vi "Renishaw-XL80_GetMatTemp.vi"(8 "error in (no error)":errorcluster, 11 "Renishaw-XL80_EMU in":refnum<class "Renishaw-XL80_EMU.lvclass">) -> (0 "error out":errorcluster, 1 "pStatus Array":i32[](array[ring]) items=["SENSOR_OK"=0, "SENSOR_BAD_READING"=1, "SENSOR_FAILED"=2, "SENSOR_NOT_CONNECTED"=4], 2 "Temperature Array":dbl[](array[numeric]), 3 "Renishaw-XL80_EMU out":refnum<class "Renishaw-XL80_EMU.lvclass">)   [LabVIEW 2024, in "Renishaw-XL80_EMU.lvclass"]
doc: "This method disconnects a client from a DX10.\n\nDefinition\nHRESULTGetMatTemp( [in] short nIndex, [out] SENSOR_STATUS_CODES *pStatus, [out, retval] double *pVal);\nParameters\nnIndex\nIdentifies the sensor to be read from. Its value should be in [1..3].\n\npStatus\nA variable that will be set to one of the SENSOR_STATUS_CODES.\n\npVal\nA variable that will be set to the material temperature reading from the specified sensor (in oC).\n\nComments\nThis method will return with an HRESULT of E_INVALIDARG if nIndex is not in [1..3].\n\nIf the client has not connected to the DX10 then the default value (20oC) will be returned and the status will be set to SENSOR_NOT_CONNECTED.\n\nIf the client connected to a DX10 and it subsequently stopped responding, or the EC10 stopped responding then the last values obtained from the EC10 will be returned i.e. the status will not be modified. It is important therefore to monitor both the DX10Status and EC10Status. This is easily done using the _RenishawDX10Events interface.\n\n\nIf the sensor status is SENSOR_NOT_CONNECTED or SENSOR_BAD_READING, then pVal will be set to the last known valid reading.\n\nThe property will normally return an HRESULT of S_OK. However, it will return E_POINTER if the client supplies a null pointer for either pVal or pStatus."
uses:
  Renishaw-XL80_EMU.lvclass
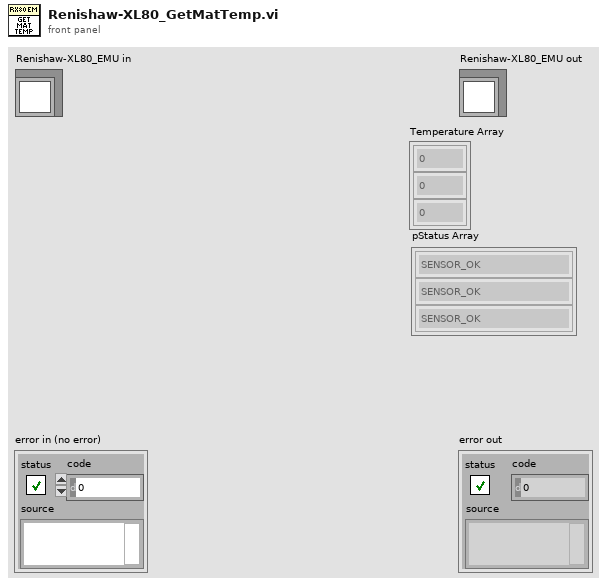
[diagram p1: front panel]
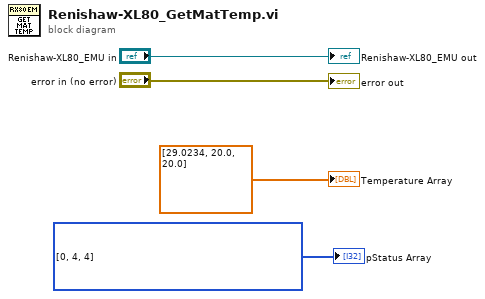
[diagram p0: block diagram]
diagram:
  w1 = i32[] [0, 4, 4] items=["SENSOR_OK"=0, "SENSOR_BAD_READING"=1, "SENSOR_FAILED"=2, "SENSOR_NOT_CONNECTED"=4] ("pStatus Array")
  "error out" <- "error in (no error)"
  "Renishaw-XL80_EMU out" <- "Renishaw-XL80_EMU in"
  "Temperature Array" <- dbl[] [29.0234, 20.0, 20.0] ("Temperature Array")
  "pStatus Array" <- w1
